vi "Write MultCol Listbox Data.vi"(8 "error in":errorcluster, 10 "Value":string[][](array[string]), 11 "Multicolumn Listbox Ref in":refnum<vi>) -> (0 "error out":errorcluster, 3 "Multicolumn Listbox Ref out":refnum<vi>)   [LabVIEW 2020, in "G-Unicode.lvlib"]
uses:
  G-Unicode.lvlib
  Unicode/Controls/String Encoding.ctl
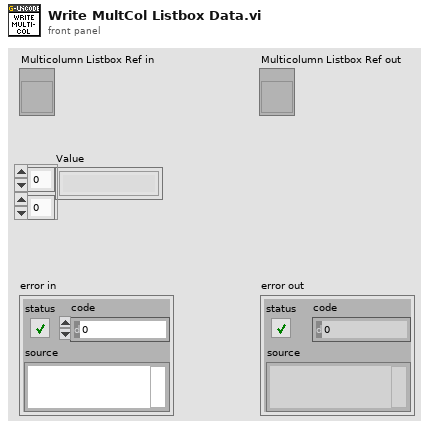
[diagram p1: front panel]
types:
  T1 = typedef "G-Unicode.lvlib/String Encoding.ctl" = enum16{"ANSI", "UTF-8", "UTF-16LE", "UTF-16BE", "Unknown"}
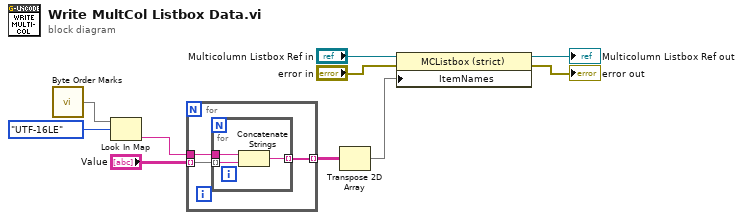
[diagram p0: block diagram]
diagram:
  n1 = call "Byte Order Marks.vi"() -> ("BOMs"=w5:map{T1, string})
  n2 = Look In Map(map=w5, key=String_Encoding."UTF-16LE") -> (value=w3:string)  [unwired: 1 in, 1 out]
  n3 = for {
    tunnel: "Value" -> [w13] mode=indexing
    tunnel: [w12] -> w6 mode=indexing
    tunnel: w3 -> [w11]
    n4 = for {
      tunnel: w13 -> [w16] mode=indexing
      tunnel: [w15] -> w12 mode=indexing
      tunnel: w11 -> [w14]
      n5 = Concatenate Strings(w14, w16) -> (w15:string)
    }
  }
  n6 = Transpose 2D Array(2D array=w6) -> (transposed array=w1:string[][])
  n7 = property class="MCListbox (strict)"(reference="Multicolumn Listbox Ref in", error in="error in", "ItemNames"=w1) -> (reference out=→"Multicolumn Listbox Ref out":refnum<vi>, error out=→"error out":errorcluster)
